vi "Create Pattern Script(OpCode).vi"(6 "Period(ms)":dbl, 8 "error in (no error)":errorcluster, 9 "String in":string, 10 "OpCode":string[](array[string]), 11 "SPI 3W Pattern Creator in":refnum<class "SPI 3W Pattern Creator.lvclass">) -> (0 "error out":errorcluster, 2 "String out":string, 3 "SPI 3W Pattern Creator out":refnum<class "SPI 3W Pattern Creator.lvclass">)   [LabVIEW 2018, in "SPI 3W Pattern Creator.lvlib" / "SPI 3W Pattern Creator.lvclass"]
uses:
  SPI 3W Pattern Creator.lvclass
  Protocols/SPI Root Pattern Creator.lvlibp/Plugins/SouceCode/SPI_Pattern Creator/SPI Root/Special Frame Type.ctl
  Interfaces/Protocol Interface.lvlibp/Interfaces/Protocol Interface/Pin State.ctl
  Interfaces/Protocol Interface.lvlibp/Interfaces/Protocol Interface/Protocol Interface.lvclass
  Protocols/SPI Root Pattern Creator.lvlibp/Plugins/SouceCode/SPI_Pattern Creator/SPI Root/SPI Root Pattern Creator.lvclass
  C:/P4 Workspace/PC Client/Solutions/5g_eap/trunk/1.0/HiSi5GmmWave/Pattern_Gen_Tool/Plugins/Protocols/SPI Root Pattern Creator.lvlibp/Plugins/SouceCode/SPI_Pattern Creator/SPI Root/SPI Root Pattern Creator.lvclass
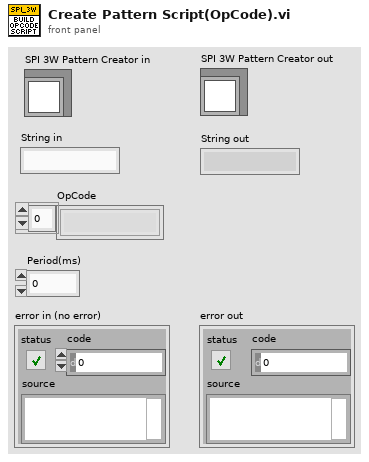
[diagram p1: front panel]
types:
  T1 = typedef "SPI Root Pattern Creator.lvlibp/SPI Root Pattern Creator.lvclass/Special Frame Type.ctl" = enum16{"SPI 4W FRM Start", "SPI 4W Wait", "SPI 4W FRM End", "SPI 4W Write Cmd", "SPI Rd Collect Cmd", "SPI Rd Value Cmd", "SPI 3W FRM Start", "SPI 3W Write Cmd", "SPI 3W FRM End", "SPI 3W Wait", "SPI 3W Rd Cmd"}
  T2 = typedef "Protocol Interface.lvlibp/Protocol Interface.lvclass/Pin State.ctl" = enum16{"0", "1", "L", "H", "X", "V", "D", "M"}
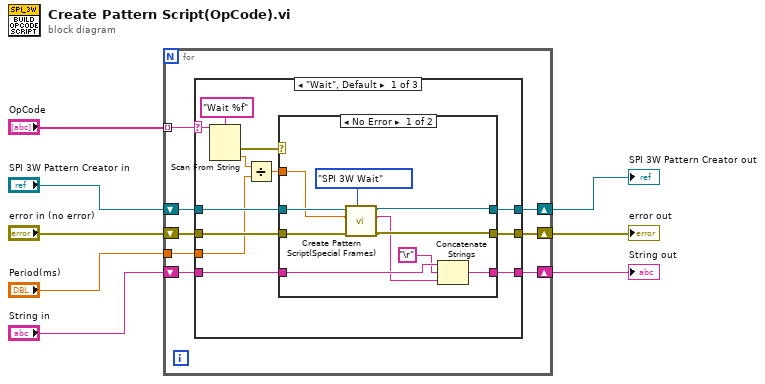
[diagram p0: block diagram]
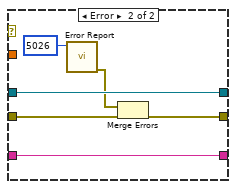
[diagram p2: hidden frame]
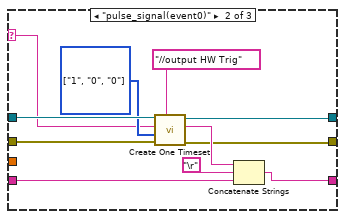
[diagram p3: hidden frame]
diagram:
  n1 = for {
    tunnel: "OpCode" -> [w16] mode=indexing
    shift-right: [w11] -> w7
    shift-left: "String in" -> [w15]
    shift-right: [w10] -> w6
    shift-left: "SPI 3W Pattern Creator in" -> [w14]
    shift-right: [w9] -> w8
    shift-left: "error in (no error)" -> [w13]
    tunnel: "Period(ms)" -> [w12]
    n2 = case shown="\"Wait\", Default" w16 {
      selector: w16 -> [w28 w51 _]
      tunnel: w15 -> [w20 w48 w56]
      tunnel: w14 -> [w25 w55 w58]
      tunnel: w13 -> [w24 w54 w57]
      tunnel: w12 -> [w21 _ _]
      tunnel: [w19 w47 w56] -> w11
      tunnel: [w18 w45 w58] -> w10
      tunnel: [w17 w46 w57] -> w9
      frame "Wait", Default {
        n3 = Scan From String(format string="Wait %f", input string=w28) -> (error out=w26:errorcluster, output 1=w22:dbl)  [unwired: 3 in, 2 out]
        n4 = Divide(x=w22, y=w21) -> (x/y=w23:dbl)
        n5 = case shown="No Error" w26 {
          tunnel: w23 -> [w33 _]
          tunnel: w25 -> [w34 w43]
          tunnel: w24 -> [w32 w44]
          tunnel: w20 -> [w38 w41]
          tunnel: [w36 w41] -> w19
          tunnel: [w35 w43] -> w18
          tunnel: [w31 w42] -> w17
          frame No Error {
            n6 = call "Create Pattern Script(Special Frames).vi"("Special Frame Type"=Special_Frame_Type."SPI 3W Wait", "error in (no error)"=w32, "Num of Timeset"=w33, "SPI Root Pattern Creator in"=w34) -> ("error out"=w31:errorcluster, "String out"=w30:string, "SPI Root Pattern Creator out"=w35:refnum<class "SPI 3W Pattern Creator.lvclass">)  [unwired: 5 in]
            n7 = Concatenate Strings(w38, "\r", w30) -> (w36:string)
          }
          frame Error {
            n8 = call "Error Report.vi"("Error Code"=i16 5026) -> ("error out"=w39:errorcluster)  [unwired: 10 in]
            n9 = Merge Errors(w39, w44) -> (w42:errorcluster)
          }
        }
      }
      frame "pulse_signal(event0)" {
        w53 = T2[] [enum."1", enum."0", enum."0"] items=["0", "1", "L", "H", "X", "V", "D", "M"] ("PinStates")
        n10 = call-dynamic "Create One Timeset.vi"("Notes"="//output HW Trig", "error in (no error)"=w54, "PinStates"=w53, "OpCode"=w51, "SPI 3W Pattern Creator in"=w55) -> ("error out"=w46:errorcluster, "String  out"=w50:string, "SPI 3W Pattern Creator out"=w45:refnum<class "SPI 3W Pattern Creator.lvclass">)  [unwired: 4 in]
        n11 = Concatenate Strings(w50, "\r", w48) -> (w47:string)
      }
      frame "" {
      }
    }
  }
  "error out" <- w8
  "String out" <- w7
  "SPI 3W Pattern Creator out" <- w6
